vi "ciclo for seno.vi"() -> ()   [LabVIEW 2020]
panel:
  out "XY Graph":cluster{dbl[], dbl[]}(graph)
  out "seno x":dbl[](array[numeric])
  out "x":dbl[](array[numeric])
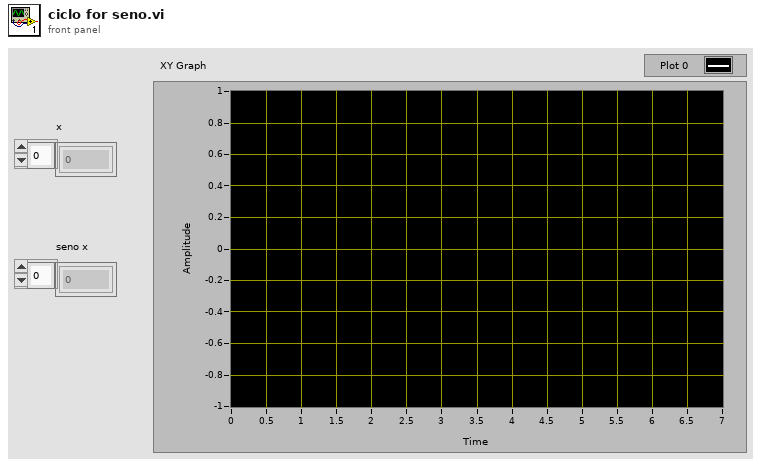
[diagram p1: front panel]
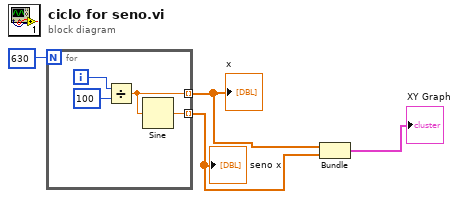
[diagram p0: block diagram]
diagram:
  n1 = for {
    N: 630 -> [_]
    tunnel: [w6] -> w2 mode=indexing
    tunnel: [w5] -> w1 mode=indexing
    i -> [w8]
    n2 = Divide(x=w8, y=100) -> (x/y=w6:dbl)
    n3 = Sine(x=w6) -> (sin(x)=w5:dbl)
  }
  "seno x" <- w1
  "x" <- w2
  n4 = Bundle(w2, w1) -> (→"XY Graph":cluster{dbl[], dbl[]})  [unwired: 1 in]
